vi "rotate.vi"(8 "error in":errorcluster, 9 "y":i32[](array[numeric]), 10 "x":i32[](array[numeric]), 11 "Data 2":T1={"App State"="", "Connect "=FALSE, "phandle out"=0, "Axis"=[], "S ramp"=30.0, "Acceleration"=100000.0, "Initial Speed"=10.0, "Normal Open / Close"=enum."Close", "Deceleration"=100000.0, "Creep"=30.0, "Speed"=1000.0, "X Axis"={"Operating State"="", "Current Position"=0.0, "Current Speed"=0.0, "Axis State"=0, "Angle"=0.0}, "Y Axis"={"Operating State"="", "Current Position"=0.0, "Current Speed"=0.0, "Axis State"=0, "Angle"=0.0}, "Distance"=0.0, "Direct of movement"=enum."Forward", "Move Method"=enum."Continue", "Move Mode"=enum."Relative", "Angle"=enum."0", "Times"=0, "Start Time"=0.0, "Step Flag"=FALSE, "x  dist"=[], "y dist"=[], "x angle array"=[], "y angle array"=[]}) -> (0 "error out 2":errorcluster, 3 "Data":T1={"App State"="", "Connect "=FALSE, "phandle out"=0, "Axis"=[], "S ramp"=30.0, "Acceleration"=100000.0, "Initial Speed"=10.0, "Normal Open / Close"=enum."Close", "Deceleration"=100000.0, "Creep"=30.0, "Speed"=1000.0, "X Axis"={"Operating State"="", "Current Position"=0.0, "Current Speed"=0.0, "Axis State"=0, "Angle"=0.0}, "Y Axis"={"Operating State"="", "Current Position"=0.0, "Current Speed"=0.0, "Axis State"=0, "Angle"=0.0}, "Distance"=0.0, "Direct of movement"=enum."Forward", "Move Method"=enum."Continue", "Move Mode"=enum."Relative", "Angle"=enum."0", "Times"=0, "Start Time"=0.0, "Step Flag"=FALSE, "x  dist"=[], "y dist"=[], "x angle array"=[], "y angle array"=[]})   [LabVIEW 2015]
uses:
  Typedef/Data2.ctl
  CUB/zauxdll-2014/zauxdll.lvlib
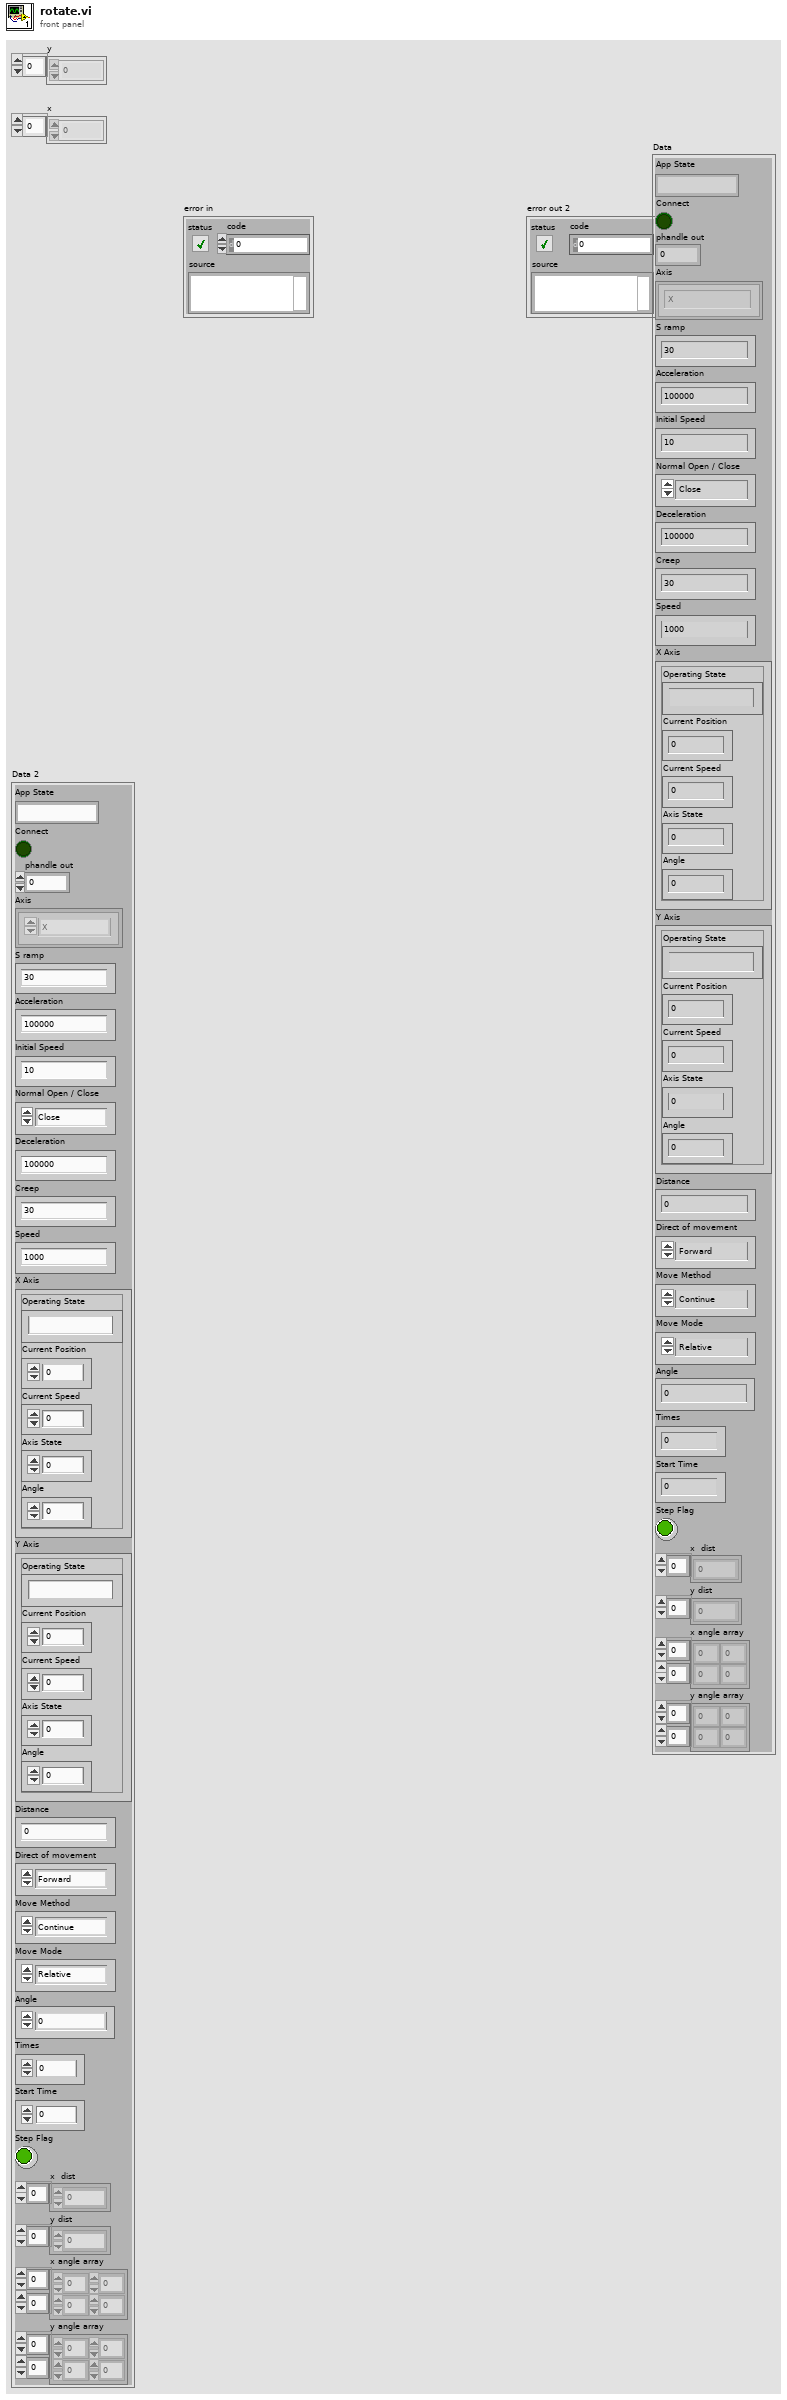
[diagram p1: front panel]
types:
  T1 = typedef "Data2.ctl" = cluster{"App State":string, "Connect ":bool, "phandle out":u32, "Axis":enum16{"X", "Y", "X+Y"}[], "S ramp":dbl, "Acceleration":dbl, "Initial Speed":dbl, "Normal Open / Close":enum16{"Open", "Close"}, "Deceleration":dbl, "Creep":dbl, "Speed":dbl, "X Axis":cluster{"Operating State":string, "Current Position":dbl, "Current Speed":dbl, "Axis State":i32, "Angle":dbl}, "Y Axis":cluster{"Operating State":string, "Current Position":dbl, "Current Speed":dbl, "Axis State":i32, "Angle":dbl}, "Distance":dbl, "Direct of movement":enum16{"Forward", "Backward"}, "Move Method":enum16{"Continue", "Inching"}, "Move Mode":enum16{"Relative", "Absolute"}, "Angle":enum32{"0", "1", "10", "30", "34", "60", "90", "180", "-1", "-10"}, "Times":i32, "Start Time":dbl, "Step Flag":bool, "x  dist":dbl[], "y dist":dbl[], "x angle array":i32[][], "y angle array":i32[][]}
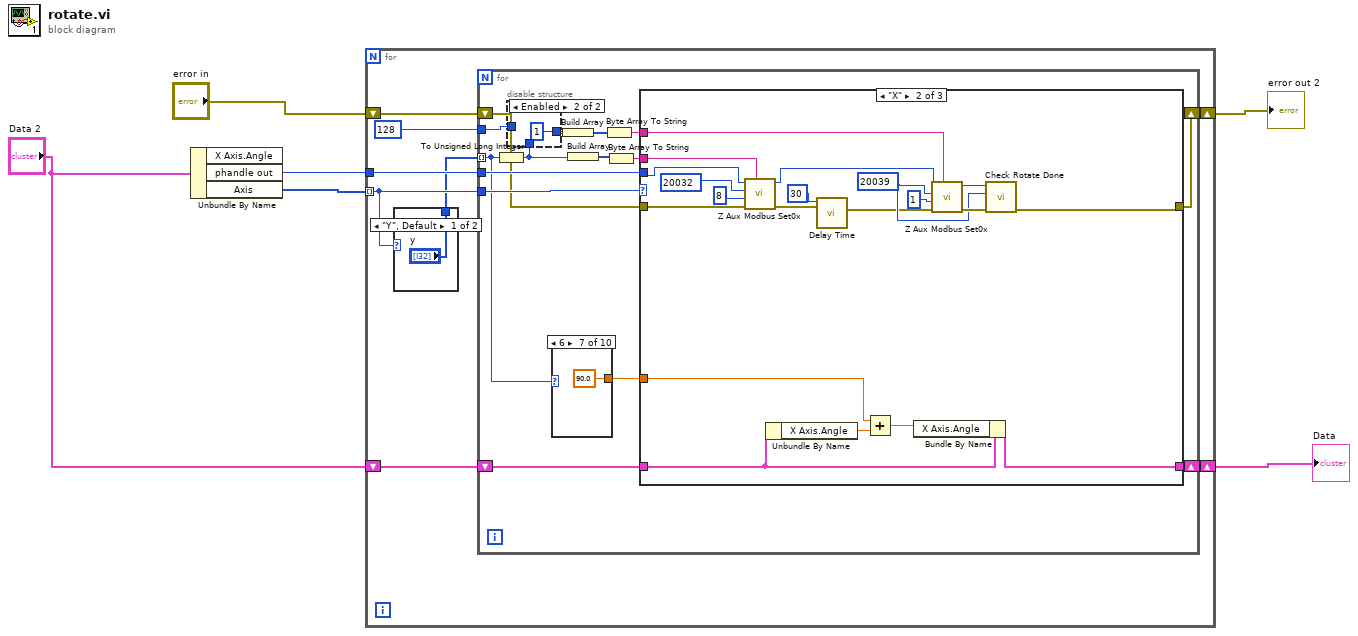
[diagram p0: block diagram]
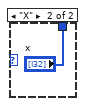
[diagram p2: hidden frame]
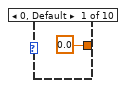
[diagram p3: hidden frame]
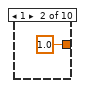
[diagram p4: hidden frame]
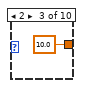
[diagram p5: hidden frame]
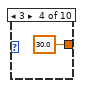
[diagram p6: hidden frame]
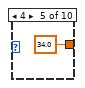
[diagram p7: hidden frame]
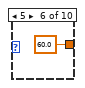
[diagram p8: hidden frame]
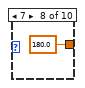
[diagram p9: hidden frame]
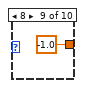
[diagram p10: hidden frame]
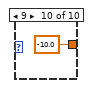
[diagram p11: hidden frame]
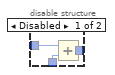
[diagram p12: hidden frame]
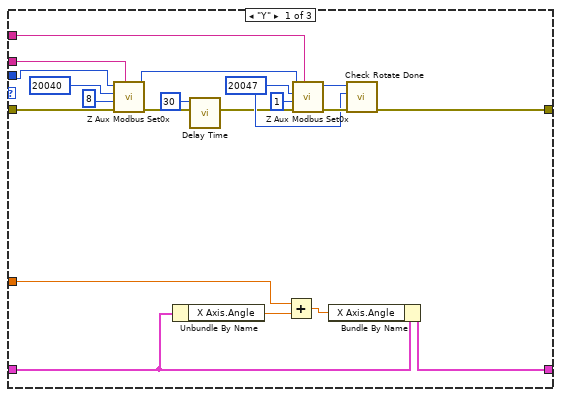
[diagram p13: hidden frame]
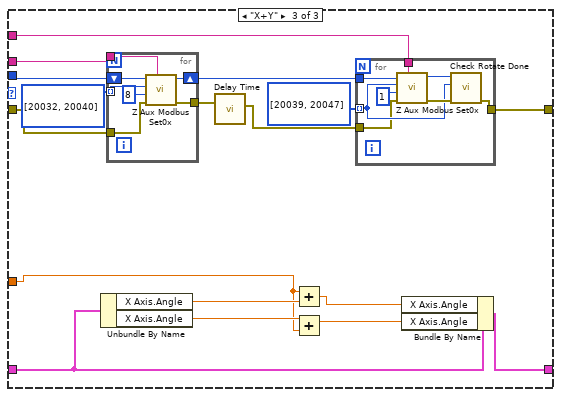
[diagram p14: hidden frame]
diagram:
  n1 = Unbundle By Name("Data 2") -> ("phandle out"=w6:u32, "Axis"=w5:enum16{"X", "Y", "X+Y"}[])  [unwired: 1 out]
  n2 = for {
    tunnel: w6 -> [w14]
    tunnel: w5 -> [w8] mode=indexing
    shift-right: [w11] -> w2
    shift-left: "error in" -> [w12]
    shift-right: [w9] -> w1
    shift-left: "Data 2" -> [w10]
    n3 = case shown="\"Y\", Default" w8 {
      tunnel: ["y" "x"] -> w7
      frame "Y", Default {
      }
      frame "X" {
      }
    }
    n4 = for {
      tunnel: w14 -> [w31]
      tunnel: w8 -> [w30]
      tunnel: u32 128 -> [w29]
      shift-right: [w22] -> w11
      shift-left: w12 -> [w23]
      shift-right: [w20] -> w9
      shift-left: w10 -> [w21]
      tunnel: w7 -> [w17] mode=indexing
      n5 = To Unsigned Long Integer(number=w17) -> (unsigned 32bit integer=w19:u32)
      n6 = disable-structure shown="Enabled" {
        disable-tunnel: w29 -> [w44 _]
        disable-tunnel: [w43 u32 1] -> w28
        disable-tunnel: w19 -> [w42 _]
        frame Disabled {
          n7 = Add(x=w44, y=w42) -> (x+y=w43:u32)
        }
        frame Enabled {
        }
      }
      n8 = case shown="6" w17 {
        tunnel: [0.0 1.0 10.0 30.0 34.0 60.0 90.0 180.0 -1.0 -10.0] -> w18
        frame 0, Default {
        }
        frame 1 {
        }
        frame 2 {
        }
        frame 3 {
        }
        frame 4 {
        }
        frame 5 {
        }
        frame 6 {
        }
        frame 7 {
        }
        frame 8 {
        }
        frame 9 {
        }
      }
      n9 = Build Array(w28) -> (w27:u32[])
      n10 = Build Array(w19) -> (w25:u32[])
      n11 = Byte Array To String(unsigned byte array=w27) -> (string=w26:string)
      n12 = Byte Array To String(unsigned byte array=w25) -> (string=w24:string)
      n13 = case shown="\"X\"" w30 {
        tunnel: w31 -> [w62 w82 w101]
        tunnel: w26 -> [w63 w83 w102]
        tunnel: w24 -> [w61 w81 w100]
        tunnel: w23 -> [w56 w76 w97]
        tunnel: [w51 w71 w93] -> w22
        tunnel: w21 -> [w50 w70 w90]
        tunnel: [w49 w69 w89] -> w20
        tunnel: w18 -> [w46 w66 w86]
        frame "Y" {
          w57 = u16 20047 ("start")
          n14 = call "Z Aux Modbus Set0x.vi"("pdata"=w61, "error in (no error)"=w56, "inum"=u16 8, "start"=u16 20040, "handle"=w62) -> ("error out"=w54:errorcluster, "handle out"=w55:u32)  [unwired: 3 in, 2 out]
          n15 = Unbundle By Name(w50) -> ("X Axis.Angle"=w47:dbl)
          n16 = call "Delay Time.vi"("error in (no error)"=w54, "Delay(ms)"=u32 30) -> ("error out"=w52:errorcluster)  [unwired: 9 in]
          n17 = Add(x=w46, y=w47) -> (x+y=w48:dbl)
          n18 = call "Z Aux Modbus Set0x.vi"("pdata"=w63, "error in (no error)"=w52, "inum"=u16 1, "start"=w57, "handle"=w55) -> ("error out"=w65:errorcluster, "handle out"=w64:u32)  [unwired: 3 in, 2 out]
          n19 = Bundle By Name(cluster=w50, "X Axis.Angle"=w48) -> (w49:T1)
          n20 = call "Check Rotate Done.vi"("error in (no error)"=w65, "start"=w57, "phandle in"=w64) -> ("error out"=w51:errorcluster)  [unwired: 8 in]
        }
        frame "X" {
          w77 = u16 20039 ("start")
          n21 = call "Z Aux Modbus Set0x.vi"("pdata"=w81, "error in (no error)"=w76, "inum"=u16 8, "start"=u16 20032, "handle"=w82) -> ("error out"=w74:errorcluster, "handle out"=w75:u32)  [unwired: 3 in, 2 out]
          n22 = Unbundle By Name(w70) -> ("X Axis.Angle"=w68:dbl)
          n23 = call "Delay Time.vi"("error in (no error)"=w74, "Delay(ms)"=u32 30) -> ("error out"=w72:errorcluster)  [unwired: 9 in]
          n24 = Add(x=w66, y=w68) -> (x+y=w67:dbl)
          n25 = Bundle By Name(cluster=w70, "X Axis.Angle"=w67) -> (w69:T1)
          n26 = call "Z Aux Modbus Set0x.vi"("pdata"=w83, "error in (no error)"=w72, "inum"=u16 1, "start"=w77, "handle"=w75) -> ("error out"=w85:errorcluster, "handle out"=w84:u32)  [unwired: 3 in, 2 out]
          n27 = call "Check Rotate Done.vi"("error in (no error)"=w85, "start"=w77, "phandle in"=w84) -> ("error out"=w71:errorcluster)  [unwired: 8 in]
        }
        frame "X+Y" {
          n28 = Unbundle By Name(w90) -> ("X Axis.Angle"=w92:dbl, "X Axis.Angle"=w91:dbl)
          n29 = for {
            tunnel: w100 -> [w116]
            shift-right: [w115] -> w95
            shift-left: w101 -> [w117]
            tunnel: i32[] [20032, 20040] -> [w113] mode=indexing
            tunnel: w97 -> [w112]
            tunnel: [w111] -> w96
            n30 = call "Z Aux Modbus Set0x.vi"("pdata"=w116, "error in (no error)"=w112, "inum"=u16 8, "start"=w113, "handle"=w117) -> ("error out"=w111:errorcluster, "handle out"=w115:u32)  [unwired: 3 in, 2 out]
          }
          n31 = call "Delay Time.vi"("error in (no error)"=w96) -> ("error out"=w94:errorcluster)  [unwired: 10 in]
          n32 = Add(x=w86, y=w92) -> (x+y=w88:dbl)
          n33 = Add(x=w91, y=w86) -> (x+y=w87:dbl)
          n34 = for {
            tunnel: w102 -> [w108]
            tunnel: w95 -> [w107]
            tunnel: i32[] [20039, 20047] -> [w105] mode=indexing
            tunnel: w94 -> [w104]
            tunnel: [w103] -> w93
            n35 = call "Z Aux Modbus Set0x.vi"("pdata"=w108, "error in (no error)"=w104, "inum"=u16 1, "start"=w105, "handle"=w107) -> ("error out"=w110:errorcluster, "handle out"=w109:u32)  [unwired: 3 in, 2 out]
            n36 = call "Check Rotate Done.vi"("error in (no error)"=w110, "start"=w105, "phandle in"=w109) -> ("error out"=w103:errorcluster)  [unwired: 8 in]
          }
          n37 = Bundle By Name(cluster=w90, "X Axis.Angle"=w88, "X Axis.Angle"=w87) -> (w89:T1)
        }
      }
    }
  }
  "error out 2" <- w2
  "Data" <- w1
